vi "CSV.vi"(0 "System no.":i32=1 min=1 max=4 step=1, 2 "Syntax":T1, 5 "error in":errorcluster) -> (14 "Controller error":bool, 19 "error out":errorcluster)   [LabVIEW 2026]
doc: "Sets GCS syntax version. Controller error is TRUE if selected system reports an error code which is not 0.\n\nE-517: GCS syntax version must be GCS 2.0. GCS 1.0 switches to E-516 compatibility mode (use E-516 GCS LabVIEW driver set instead when working in E-516 compatibility mode). Requires command level 1, see CCL.vi.\n\nC-887, F-206, M-8X0: Only for combinations of mechanics and C-887 controller."
uses:
  Communication/Syntax.ctl
  Communication/Global1.vi
panel:
  # "Sets GCS syntax version and writes it into Global 1.vi\nif Controller error is FALSE."
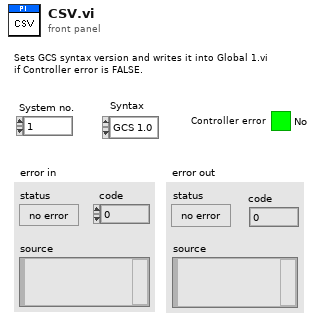
[diagram p1: front panel]
types:
  T1 = typedef "Syntax.ctl" = enum16{"GCS 1.0", "GCS 2.0", "GCS 3.0"}
  T2 = enum16{"Disable error check", "Force error check", "Use global settings"}
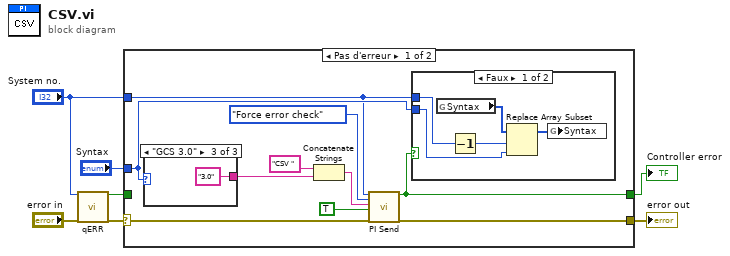
[diagram p0: block diagram]
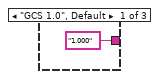
[diagram p2: hidden frame]
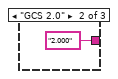
[diagram p3: hidden frame]
diagram:
  n1 = call "qERR.vi"("System no."="System no.", "error in"="error in") -> ("Controller error"=w1:bool, "error out"=w4:errorcluster)  [unwired: 16 out]
  n2 = case shown="Pas d'erreur" w4 {
    selector: w4 -> [w8 w26]
    tunnel: "Syntax" -> [w14 _]
    tunnel: "System no." -> [w12 _]
    tunnel: [w11 w26] -> w3
    tunnel: [w10 w27] -> w2
    tunnel: w1 -> [_ w27]
    frame No Error {
      n3 = case shown="\"GCS 3.0\"" w14 {
        tunnel: ["1.000" "2.000" "3.0"] -> w13
        frame "GCS 1.0", Default {
        }
        frame "GCS 2.0" {
        }
        frame "GCS 3.0" {
        }
      }
      n4 = Concatenate Strings("CSV ", w13) -> (w15:string)
      n5 = call "PI Send.vi"("System no."=w12, "Error check settings"=T2."Force error check", "String to send"=w15, "Attach termination char.?"=TRUE ("Attach Linefeed?"), "error in"=w8) -> ("Controller error"=w10:bool, "error out"=w11:errorcluster)  [unwired: 1 in, 12 out]
      n6 = case shown="Faux" w10 {
        tunnel: w12 -> [w24 _]
        tunnel: w14 -> [w22 _]
        frame False {
          n7 = global read "Global1.vi" "Syntax"() -> (w25:T1[])
          n8 = Decrement(x=w24) -> (x-1=w23:i32)
          n9 = Replace Array Subset(array=w25, new element=w22, index=w23) -> (w21:T1[])
          n10 = global write "Global1.vi" "Syntax"(w21) -> ()
        }
        frame True {
        }
      }
    }
    frame Error {
    }
  }
  "error out" <- w3
  "Controller error" <- w2
